vi "一体站流程质控自动启动.vi"(6 "CODMn量程切换":enum32{"H", "L", "AUTO"}(ring)=enum."AUTO", 8 "总磷量程切换":enum32{"H", "L", "AUTO"}(ring)=enum."AUTO", 9 "总氮量程切换":enum32{"H", "L", "AUTO"}(ring)=enum."AUTO", 10 "氨氮量程切换":enum32{"H", "L", "AUTO"}(ring)=enum."AUTO", 11 "参数":T1={"是否启用仪器"=FALSE, "CODMn"={"启动测量模式"={"测量模式"=enum."水样测量"}, "确定按钮"=TRUE}, "启动模块"={"氨氮"=FALSE, "总磷"=FALSE, "总氮"=FALSE, "CODMn"=FALSE, "CODCr"=FALSE}, "常规启动"=FALSE, "直接启动"=FALSE}) -> ()   [LabVIEW 2016, in "质控单元.lvlib"]
panel:
  out "枚举 2":enum16{"初始化", "采配水启动", "等待", "配水", "排水", "结束"}(ring)
  out "枚举":enum16{"初始化", "采配水启动", "等待", "配水", "排水", "结束"}(ring)
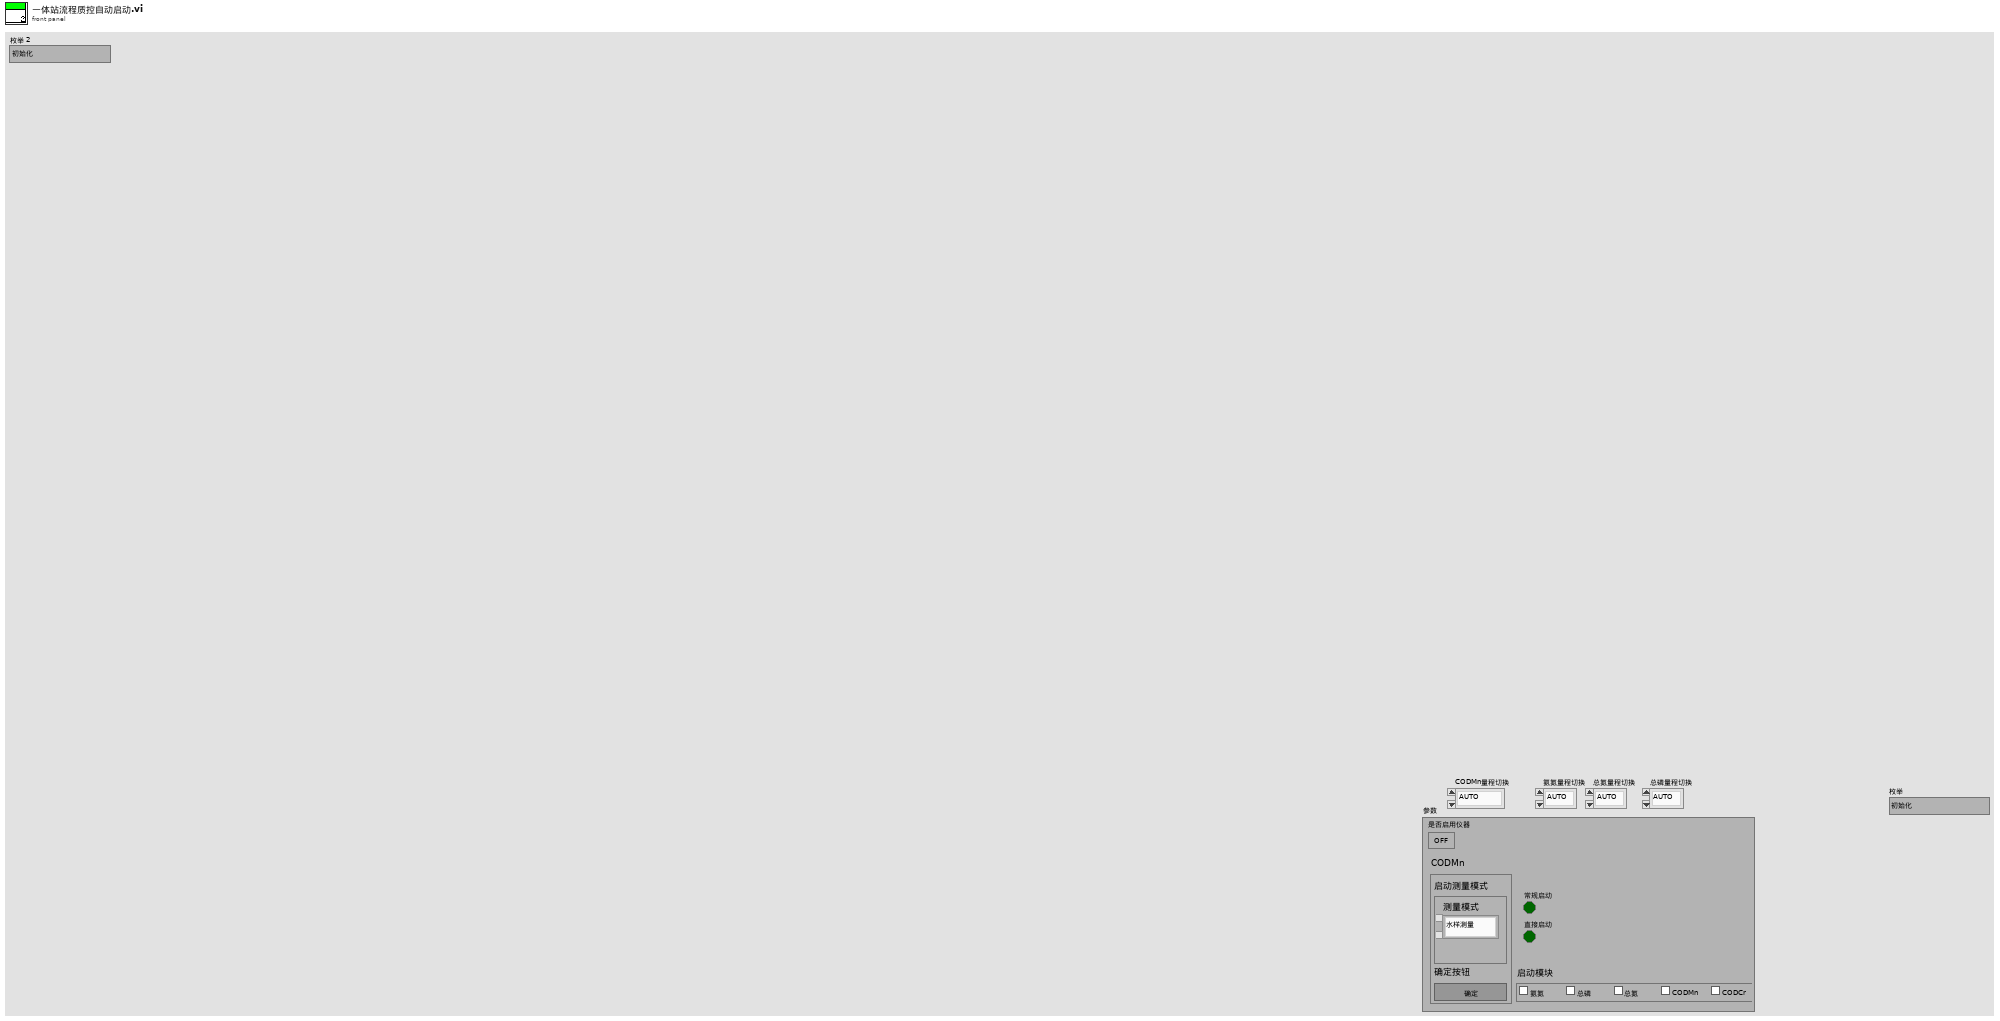
[diagram p1: front panel]
types:
  T1 = cluster{"是否启用仪器":bool, "CODMn":cluster{"启动测量模式":cluster{"测量模式":enum16{"水样测量", "标样核查", "加标回收", "平行样", "校零", "校标"}}, "确定按钮":bool}, "启动模块":cluster{"氨氮":bool, "总磷":bool, "总氮":bool, "CODMn":bool, "CODCr":bool}, "常规启动":bool, "直接启动":bool}
  T2 = cluster{"命令":string, cluster{"starting address":u16, "holding register value":u16}}
  T3 = cluster{"R0":i16, "R1":i16, "R2":i16, "R3":i16, "R4":i16, "R5":i16, "R6":i16, "R7":i16, "R8":i16, "R9":i16, "R10":i16, "R11":i16, "R12":i16, "R13":i16, "R14":i16, "R15":i16, "R16":i16, "R17":i16, "R18":i16, "R19":i16, "R20":i16, "R21":i16, "R22":i16, "R23":i16, "R24":i16, "R25":i16, "R26":i16, "R27":i16, "R28":i16, "R29":i16, "R30":i16, "R31":i16, "R32":i16, "R33":i16, "R34":i16, "R35":i16, "R36":i16, "R37":i16, "R38":i16, "R39":i16, "R40":i16, "R41":i16, "R42":i16, "R43":i16, "R44":i16, "R45":i16, "R46":i16, "R47":i16, "R48":i16, "R49":i16, "R50":i16, "R51":i16, "R52":i16, "R53":i16, "R54":i16, "R55":i16, "R56":i16}
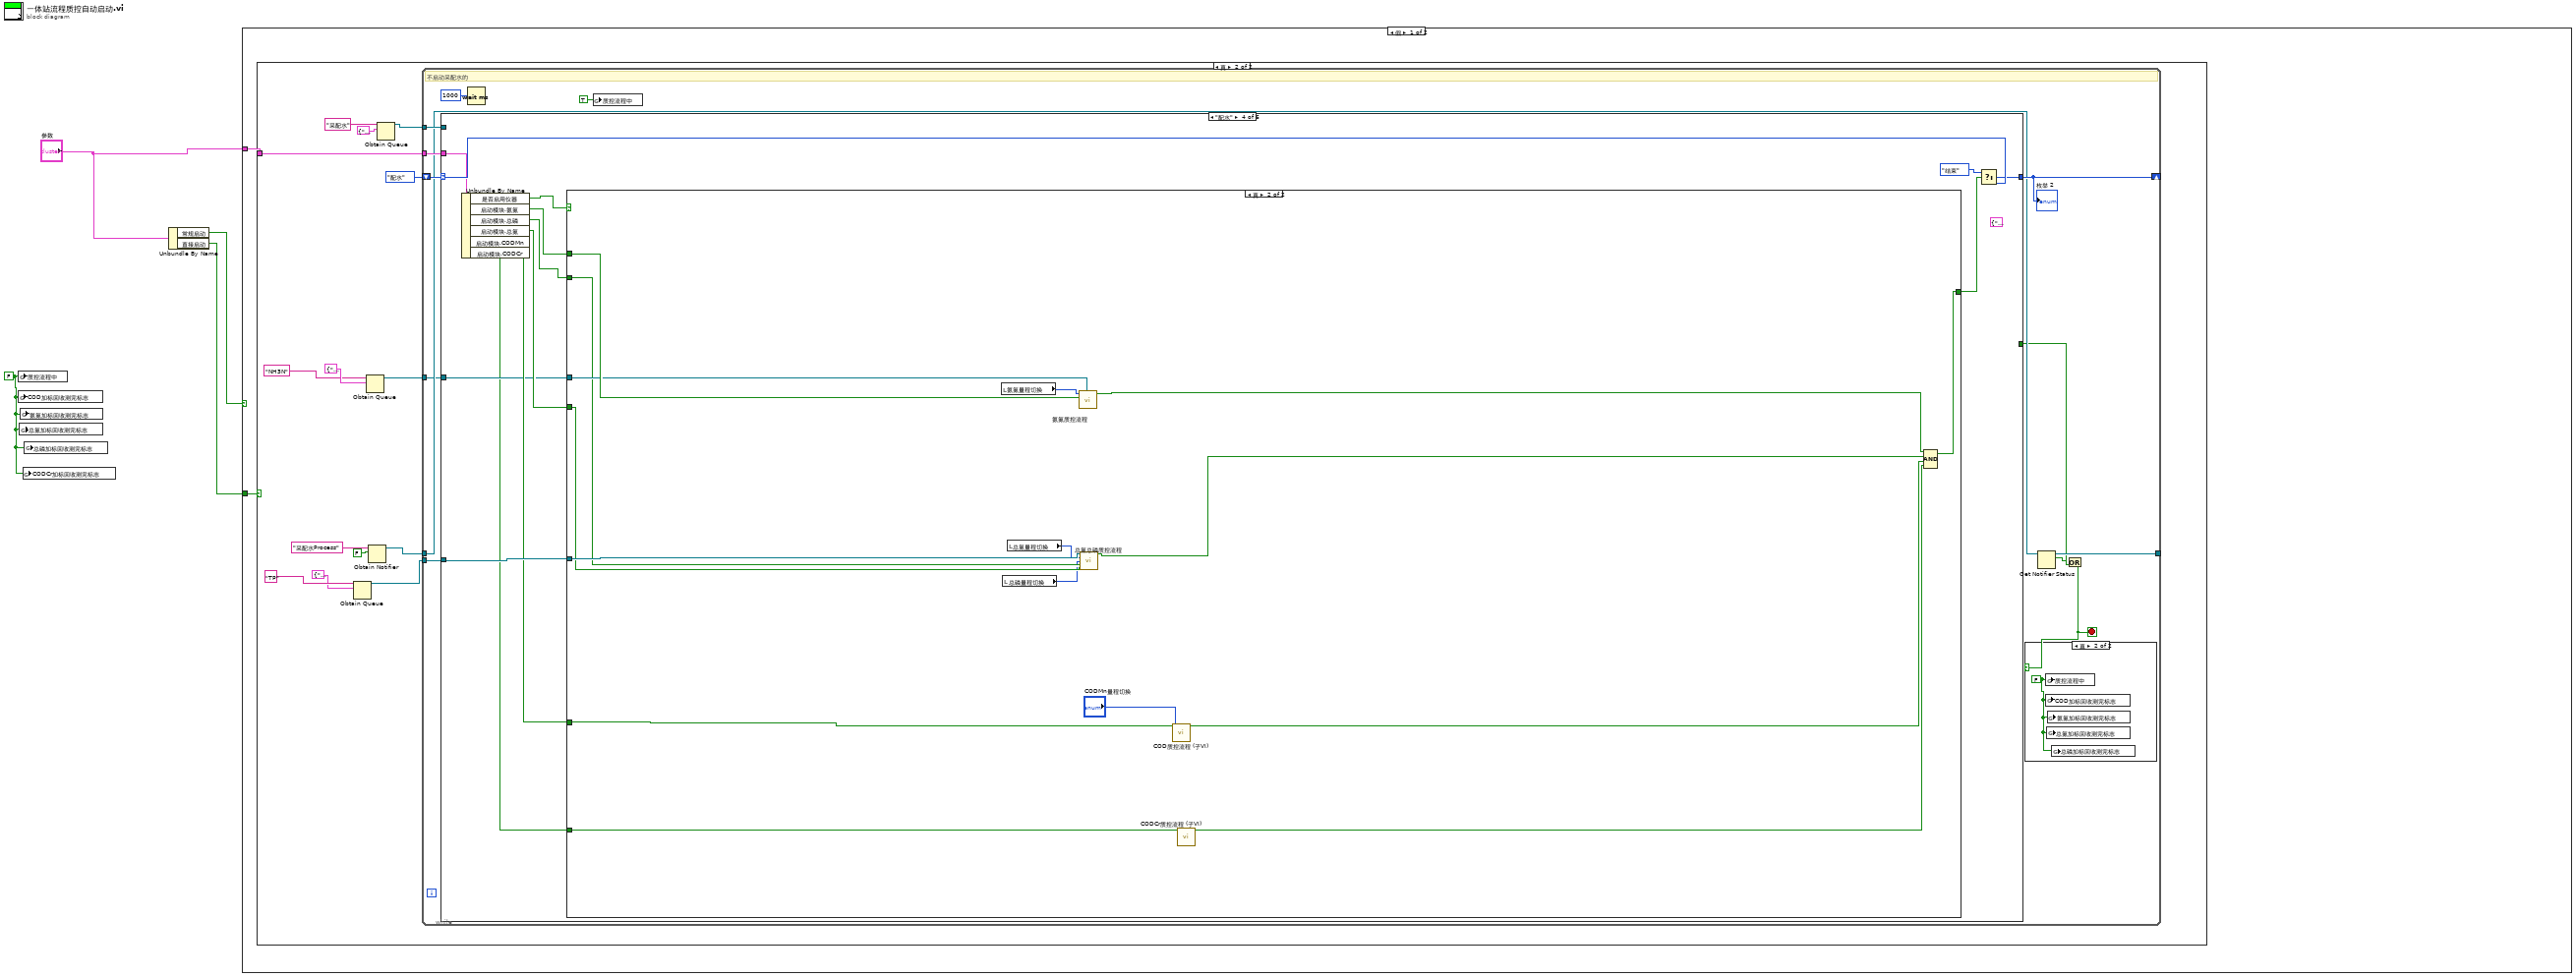
[diagram p0: block diagram]
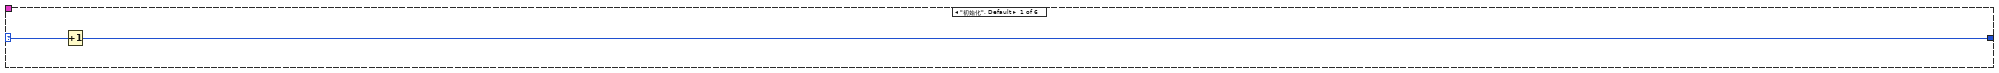
[diagram p4: hidden frame]
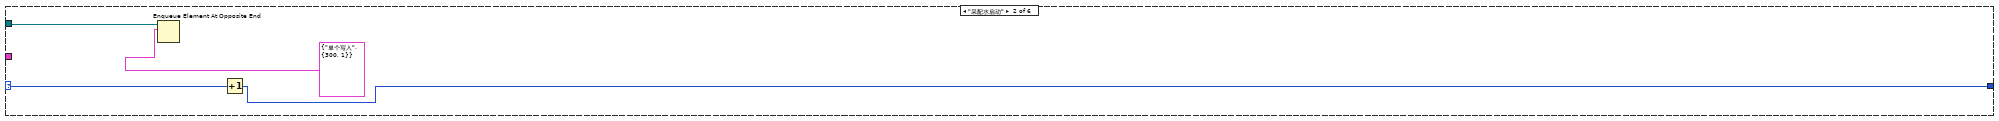
[diagram p5: hidden frame]
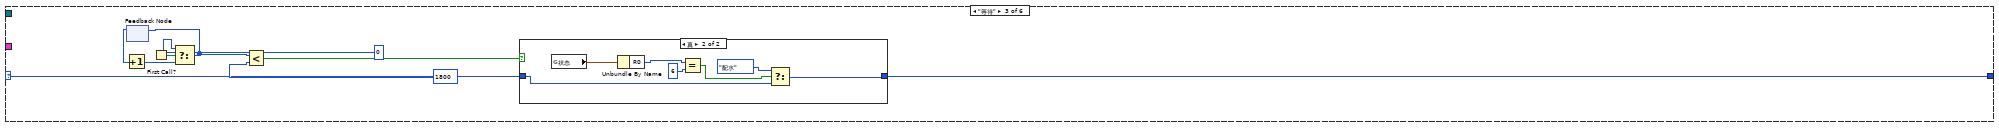
[diagram p6: hidden frame]
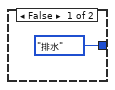
[diagram p7: hidden frame]
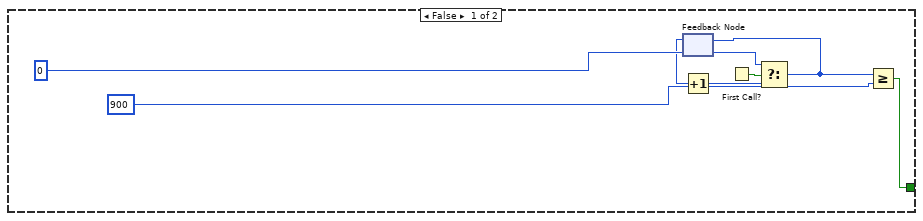
[diagram p8: hidden frame]
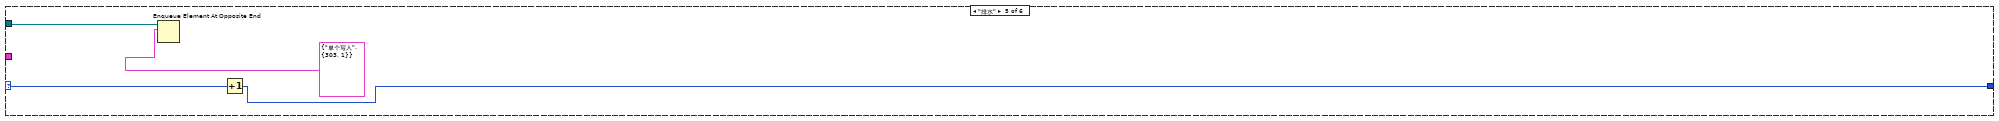
[diagram p9: hidden frame]
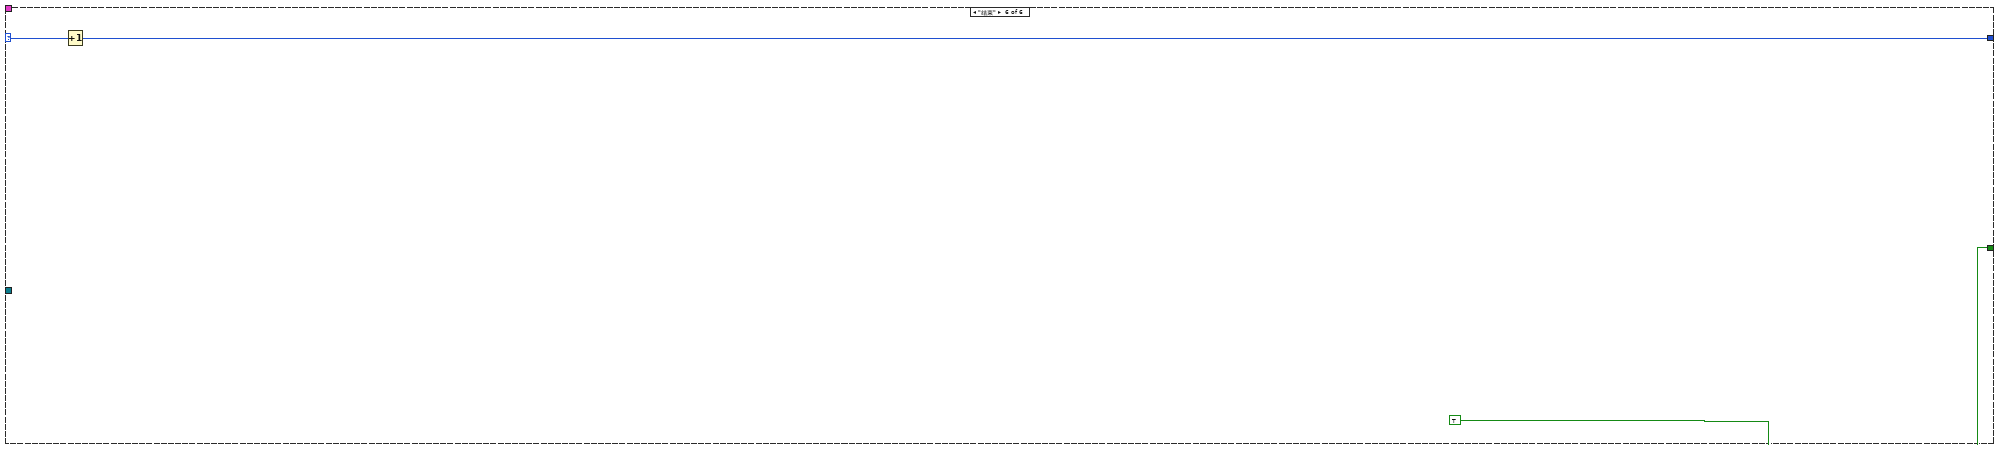
[diagram p10: hidden frame]
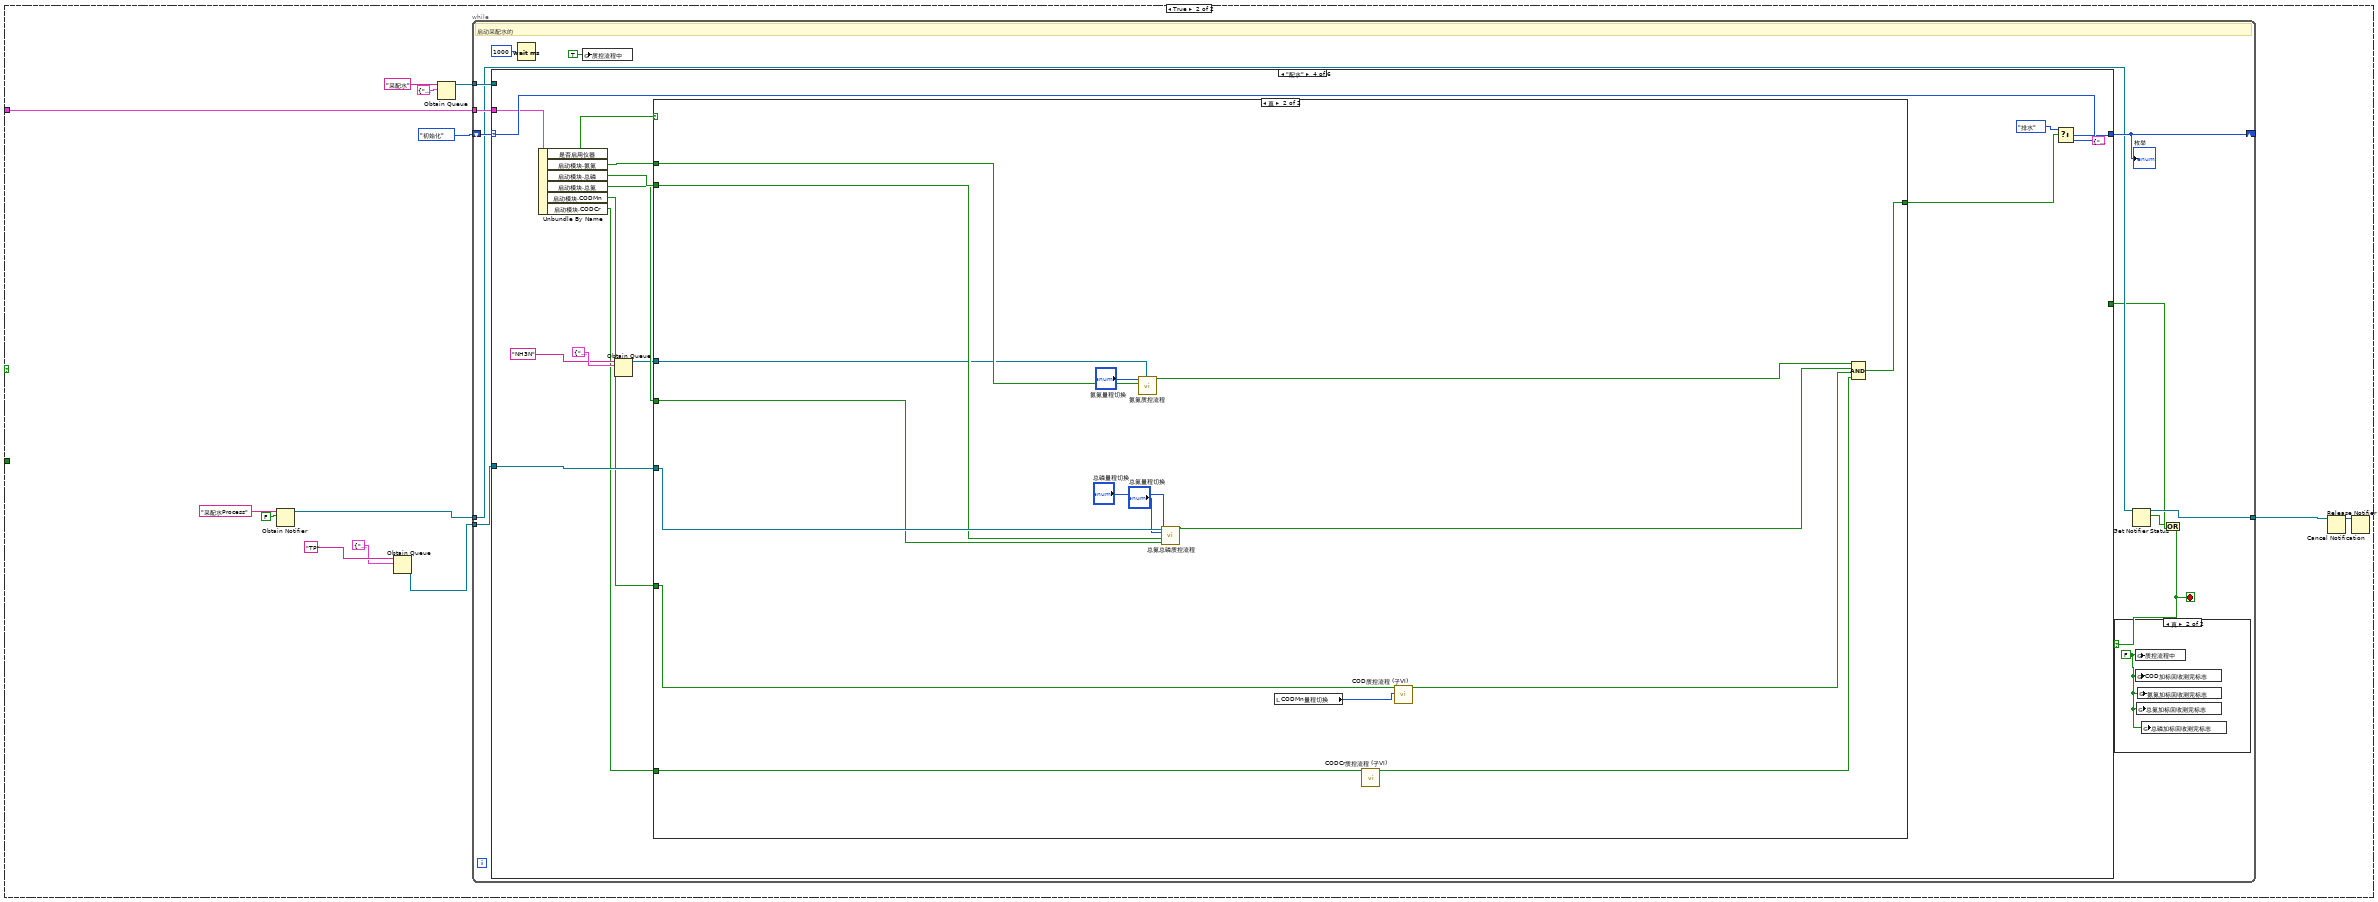
[diagram p11: hidden frame]
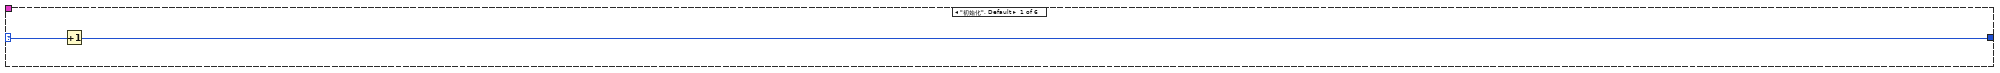
[diagram p13: hidden frame]
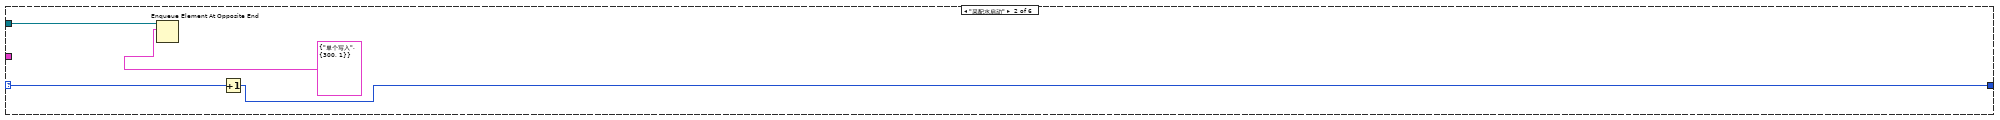
[diagram p14: hidden frame]
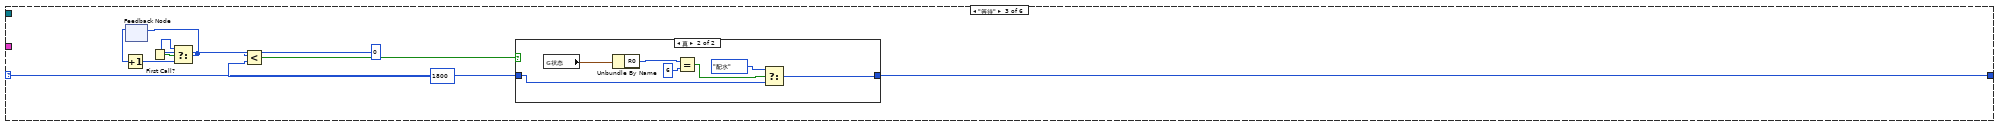
[diagram p15: hidden frame]
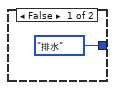
[diagram p16: hidden frame]
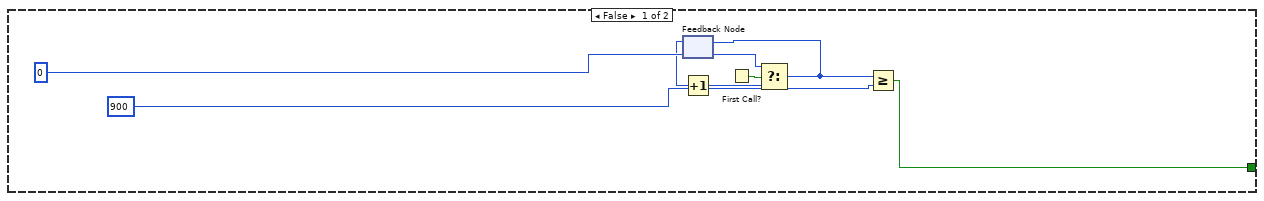
[diagram p17: hidden frame]
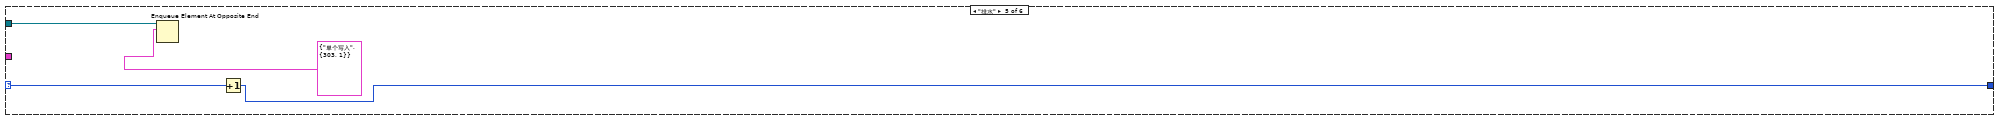
[diagram p18: hidden frame]
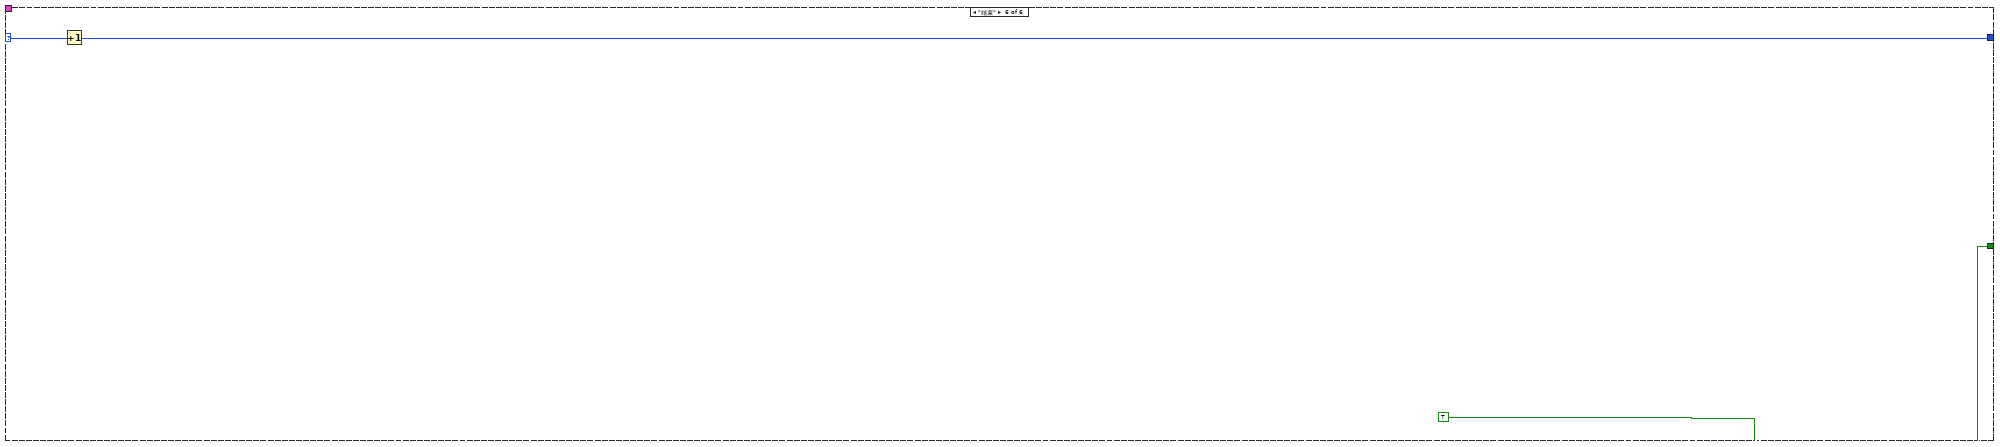
[diagram p19: hidden frame]
diagram:
  w1 = FALSE ("质控流程中")
  n1 = global write "质控测完标志全局 1.vi" "质控流程中"(w1) -> ()
  n2 = global write "质控测完标志全局 1.vi" "COD加标回收测完标志"(w1) -> ()
  n3 = global write "质控测完标志全局 1.vi" "总氮加标回收测完标志"(w1) -> ()
  n4 = global write "质控测完标志全局 1.vi" "氨氮加标回收测完标志"(w1) -> ()
  n5 = global write "质控测完标志全局 1.vi" "CODCr加标回收测完标志"(w1) -> ()
  n6 = global write "质控测完标志全局 1.vi" "总磷加标回收测完标志"(w1) -> ()
  n7 = Unbundle By Name("参数") -> ("常规启动"=w3:bool, "直接启动"=w2:bool)
  n8 = case shown="假" w3 {
    tunnel: "参数" -> [w5 w101]
    tunnel: w2 -> [w6 _]
    frame False {
      n9 = case shown="真" w6 {
        tunnel: w5 -> [_ w19]
        frame False {
        }
        frame True {
          n10 = Obtain Queue(name (unnamed)="TP" ("名称（未命名）"), element data type=cluster{"命令":string, "data":variant} {"命令"="", "data"=variant}) -> (queue out=w10:refnum<queue>)  [unwired: 3 in, 2 out]
          n11 = Obtain Queue(name (unnamed)="NH3N" ("名称（未命名）"), element data type=cluster{"命令":string, "data":variant} {"命令"="", "data"=variant}) -> (queue out=w7:refnum<queue>)  [unwired: 3 in, 2 out]
          n12 = Obtain Notifier(name (unnamed)="采配水Process" ("名称（未命名）"), notification data type=FALSE) -> (notifier out=w13:refnum<notifier>)  [unwired: 2 in, 2 out]
          n13 = Obtain Queue(name (unnamed)="采配水" ("名称（未命名）"), element data type=cluster{"命令":string, "数据":variant} {"命令"="", "数据"=variant}) -> (queue out=w16:refnum<queue>)  [unwired: 3 in, 2 out]
          n14 = while {
            tunnel: w16 -> [w33]
            shift-right: [w31] -> _
            shift-left: enum16{"初始化", "采配水启动", "等待", "配水", "排水", "结束"}."配水" ("枚举") -> [w32]
            tunnel: w10 -> [w29]
            tunnel: w19 -> [w28]
            tunnel: w13 -> [w27]
            tunnel: [w26] -> _
            tunnel: w7 -> [w23]
            stop <- w22 stop-if-true
            # "不启动采配水的"
            n15 = case shown="\"配水\"" w32 {
              selector: w32 -> [w36 w38 w47 w69 w95 w100]
              tunnel: w33 -> [_ w39 _ _ w96 _]
              tunnel: [w35 w37 w46 w68 w94 w99] -> w31
              tunnel: [_ _ _ _ _ TRUE] -> w25
              tunnel: w29 -> [_ _ _ w67 _ _]
              tunnel: w28 -> [_ _ _ w64 _ _]
              tunnel: w23 -> [_ _ _ w59 _ _]
              frame "初始化", Default {
                n16 = Increment(x=w36) -> (x+1=w35:enum16{"初始化", "采配水启动", "等待", "配水", "排水", "结束"})
              }
              frame "采配水启动" {
                n17 = Enqueue Element At Opposite End(queue=w39, element=T2 {"命令"="单个写入", {"starting address"=300, "holding register value"=1}} ("元素")) -> ()  [unwired: 2 in, 3 out]
                n18 = Increment(x=w38) -> (x+1=w37:enum16{"初始化", "采配水启动", "等待", "配水", "排水", "结束"})
              }
              frame "等待" {
                n19 = feedback #1() -> (w43:i32)  [unwired: 1 in]
                n20 = Increment(x=w43) -> (x+1=w42:i32)
                n21 = First Call?() -> (First Call?: T/F=w44:bool)
                n22 = Select(t=0, s=w44, f=w42) -> (s? t:f=w41:i32)
                n23 = feedback-in #1(w41) -> ()
                n24 = Less?(x=w41, y=1800) -> (x < y?=w48:bool)
                n25 = case shown="真" w48 {
                  tunnel: w47 -> [_ w53]
                  tunnel: [enum16{"初始化", "采配水启动", "等待", "配水", "排水", "结束"}."排水" ("枚举") w52] -> w46
                  frame False {
                  }
                  frame True {
                    n26 = global read "与采配水交互全局.vi" "状态"() -> (w51:T3)
                    n27 = Unbundle By Name(w51) -> ("R0"=w57:i16)
                    n28 = Equal?(x=w57, y=i16 6) -> (x = y?=w55:bool)
                    n29 = Select(t=enum16{"初始化", "采配水启动", "等待", "配水", "排水", "结束"}."配水" ("枚举"), s=w55, f=w53) -> (s? t:f=w52:enum16{"初始化", "采配水启动", "等待", "配水", "排水", "结束"})
                  }
                }
              }
              frame "配水" {
                (unwired) cluster{"命令":string, "data":variant} {"命令"="启动", "data"=variant(cluster{"站号":u16, "控制命令输出":u16[]} {"站号"=1, "控制命令输出"=[256, 0]})} ("元素")
                n30 = Unbundle By Name(w64) -> ("是否启用仪器"=w66:bool, "启动模块.氨氮"=w62:bool, "启动模块.总磷"=w63:bool, "启动模块.总氮"=w60:bool, "启动模块.CODMn"=w61:bool, "启动模块.CODCr"=w58:bool)
                n31 = case shown="真" w66 {
                  tunnel: w67 -> [_ w87]
                  tunnel: [w71 w93] -> w65
                  tunnel: w63 -> [_ w86]
                  tunnel: w62 -> [_ w92]
                  tunnel: w61 -> [_ w91]
                  tunnel: w60 -> [_ w85]
                  tunnel: w59 -> [_ w89]
                  tunnel: w58 -> [_ w79]
                  frame False {
                    n32 = feedback #2() -> (w75:i32)  [unwired: 1 in]
                    n33 = Increment(x=w75) -> (x+1=w74:i32)
                    n34 = First Call?() -> (First Call?: T/F=w76:bool)
                    n35 = Select(t=0, s=w76, f=w74) -> (s? t:f=w72:i32)
                    n36 = feedback-in #2(w72) -> ()
                    n37 = Greater Or Equal?(x=w72, y=900) -> (x >= y?=w71:bool)
                  }
                  frame True {
                    n38 = local read "氨氮量程切换"() -> (w80:enum32{"H", "L", "AUTO"})
                    n39 = local read "总磷量程切换"() -> (w82:enum32{"H", "L", "AUTO"})
                    n40 = local read "总氮量程切换"() -> (w81:enum32{"H", "L", "AUTO"})
                    n41 = call "氨氮质控流程.vi"("队列输入NH3"=w89, "氨氮"=w92, "氨氮量程切换"=w80) -> ("布尔"=w90:bool)  [unwired: 7 in, 1 out]
                    n42 = call "总氮总磷质控流程.vi"("队列输入TP"=w87, "总氮量程切换"=w81, "总磷量程切换"=w82, "总磷"=w86, "总氮"=w85) -> ("布尔"=w84:bool)  [unwired: 8 in, 2 out]
                    n43 = call "COD质控流程 (子VI).vi"("CODMn量程切换"="CODMn量程切换", "COD"=w91) -> ("布尔"=w88:bool)  [unwired: 8 in, 1 out]
                    n44 = call "CODCr质控流程 (子VI).vi"("CODCr"=w79) -> ("布尔"=w78:bool)  [unwired: 9 in, 1 out]
                    n45 = Compound Arithmetic op=AND ("复合运算")(w90, w84, w88, w78) -> (w93:bool)
                  }
                }
                n46 = Select(t=enum16{"初始化", "采配水启动", "等待", "配水", "排水", "结束"}."结束" ("枚举"), s=w65, f=w69) -> (s? t:f=w68:enum16{"初始化", "采配水启动", "等待", "配水", "排水", "结束"})
              }
              frame "排水" {
                n47 = Enqueue Element At Opposite End(queue=w96, element=T2 {"命令"="单个写入", {"starting address"=303, "holding register value"=1}} ("元素")) -> ()  [unwired: 2 in, 3 out]
                n48 = Increment(x=w95) -> (x+1=w94:enum16{"初始化", "采配水启动", "等待", "配水", "排水", "结束"})
              }
              frame "结束" {
                n49 = Increment(x=w100) -> (x+1=w99:enum16{"初始化", "采配水启动", "等待", "配水", "排水", "结束"})
              }
            }
            "枚举 2" <- w31
            n50 = Wait (ms)(milliseconds to wait=u32 1000 ("等待时间（毫秒）")) -> ()  [unwired: 1 out]
            n51 = global write "质控测完标志全局 1.vi" "质控流程中"(TRUE ("质控流程中")) -> ()
            n52 = Get Notifier Status(notifier=w27) -> (notifier out=w26:refnum<notifier>, current notification=w24:bool)  [unwired: 1 in, 3 out]
            n53 = Or(x=w24, y=w25) -> (x .or. y?=w22:bool)
            n54 = case shown="真" w22 {
              frame False {
              }
              frame True {
                w34 = FALSE ("质控流程中")
                n55 = global write "质控测完标志全局 1.vi" "质控流程中"(w34) -> ()
                n56 = global write "质控测完标志全局 1.vi" "COD加标回收测完标志"(w34) -> ()
                n57 = global write "质控测完标志全局 1.vi" "总氮加标回收测完标志"(w34) -> ()
                n58 = global write "质控测完标志全局 1.vi" "氨氮加标回收测完标志"(w34) -> ()
                n59 = global write "质控测完标志全局 1.vi" "总磷加标回收测完标志"(w34) -> ()
              }
            }
          }
        }
      }
    }
    frame True {
      n60 = Obtain Notifier(name (unnamed)="采配水Process" ("名称（未命名）"), notification data type=FALSE) -> (notifier out=w104:refnum<notifier>)  [unwired: 2 in, 2 out]
      n61 = Obtain Queue(name (unnamed)="TP" ("名称（未命名）"), element data type=cluster{"命令":string, "data":variant} {"命令"="", "data"=variant}) -> (queue out=w107:refnum<queue>)  [unwired: 3 in, 2 out]
      n62 = Obtain Queue(name (unnamed)="采配水" ("名称（未命名）"), element data type=cluster{"命令":string, "数据":variant} {"命令"="", "数据"=variant}) -> (queue out=w111:refnum<queue>)  [unwired: 3 in, 2 out]
      n63 = while {
        tunnel: w111 -> [w125]
        shift-right: [w123] -> _
        shift-left: enum16{"初始化", "采配水启动", "等待", "配水", "排水", "结束"}."初始化" ("枚举") -> [w124]
        tunnel: w107 -> [w121]
        tunnel: w101 -> [w120]
        tunnel: w104 -> [w119]
        tunnel: [w118] -> w103
        stop <- w115 stop-if-true
        # "启动采配水的"
        n64 = case shown="\"配水\"" w124 {
          selector: w124 -> [w128 w130 w139 w163 w189 w194]
          tunnel: w125 -> [_ w131 _ _ w190 _]
          tunnel: [w127 w129 w138 w162 w188 w193] -> w123
          tunnel: [_ _ _ _ _ TRUE] -> w117
          tunnel: w121 -> [_ _ _ w161 _ _]
          tunnel: w120 -> [_ _ _ w158 _ _]
          frame "初始化", Default {
            n65 = Increment(x=w128) -> (x+1=w127:enum16{"初始化", "采配水启动", "等待", "配水", "排水", "结束"})
          }
          frame "采配水启动" {
            n66 = Enqueue Element At Opposite End(queue=w131, element=T2 {"命令"="单个写入", {"starting address"=300, "holding register value"=1}} ("元素")) -> ()  [unwired: 2 in, 3 out]
            n67 = Increment(x=w130) -> (x+1=w129:enum16{"初始化", "采配水启动", "等待", "配水", "排水", "结束"})
          }
          frame "等待" {
            n68 = feedback #3() -> (w135:i32)  [unwired: 1 in]
            n69 = Increment(x=w135) -> (x+1=w134:i32)
            n70 = First Call?() -> (First Call?: T/F=w136:bool)
            n71 = Select(t=0, s=w136, f=w134) -> (s? t:f=w133:i32)
            n72 = feedback-in #3(w133) -> ()
            n73 = Less?(x=w133, y=1800) -> (x < y?=w140:bool)
            n74 = case shown="真" w140 {
              tunnel: w139 -> [_ w145]
              tunnel: [enum16{"初始化", "采配水启动", "等待", "配水", "排水", "结束"}."排水" ("枚举") w144] -> w138
              frame False {
              }
              frame True {
                n75 = global read "与采配水交互全局.vi" "状态"() -> (w143:T3)
                n76 = Unbundle By Name(w143) -> ("R0"=w149:i16)
                n77 = Equal?(x=w149, y=i16 6) -> (x = y?=w147:bool)
                n78 = Select(t=enum16{"初始化", "采配水启动", "等待", "配水", "排水", "结束"}."配水" ("枚举"), s=w147, f=w145) -> (s? t:f=w144:enum16{"初始化", "采配水启动", "等待", "配水", "排水", "结束"})
              }
            }
          }
          frame "配水" {
            (unwired) cluster{"命令":string, "data":variant} {"命令"="启动", "data"=variant(cluster{"站号":u16, "控制命令输出":u16[]} {"站号"=1, "控制命令输出"=[256, 0]})} ("元素")
            n79 = Unbundle By Name(w158) -> ("是否启用仪器"=w160:bool, "启动模块.氨氮"=w156:bool, "启动模块.总磷"=w157:bool, "启动模块.总氮"=w154:bool, "启动模块.CODMn"=w155:bool, "启动模块.CODCr"=w150:bool)
            n80 = Obtain Queue(name (unnamed)="NH3N" ("名称（未命名）"), element data type=cluster{"命令":string, "data":variant} {"命令"="", "data"=variant}) -> (queue out=w151:refnum<queue>)  [unwired: 3 in, 2 out]
            n81 = case shown="真" w160 {
              tunnel: w161 -> [_ w182]
              tunnel: [w165 w186] -> w159
              tunnel: w157 -> [_ w181]
              tunnel: w156 -> [_ w185]
              tunnel: w155 -> [_ w184]
              tunnel: w154 -> [_ w180]
              tunnel: w151 -> [_ w178]
              tunnel: w150 -> [_ w173]
              frame False {
                n82 = feedback #4() -> (w169:i32)  [unwired: 1 in]
                n83 = Increment(x=w169) -> (x+1=w168:i32)
                n84 = First Call?() -> (First Call?: T/F=w170:bool)
                n85 = Select(t=0, s=w170, f=w168) -> (s? t:f=w166:i32)
                n86 = feedback-in #4(w166) -> ()
                n87 = Greater Or Equal?(x=w166, y=900) -> (x >= y?=w165:bool)
              }
              frame True {
                n88 = call "氨氮质控流程.vi"("队列输入NH3"=w178, "氨氮"=w185, "氨氮量程切换"="氨氮量程切换") -> ("布尔"=w187:bool)  [unwired: 7 in, 1 out]
                n89 = call "总氮总磷质控流程.vi"("队列输入TP"=w182, "总氮量程切换"="总氮量程切换", "总磷量程切换"="总磷量程切换", "总磷"=w181, "总氮"=w180) -> ("布尔"=w179:bool)  [unwired: 8 in, 2 out]
                n90 = local read "CODMn量程切换"() -> (w177:enum32{"H", "L", "AUTO"})
                n91 = call "CODCr质控流程 (子VI).vi"("CODCr"=w173) -> ("布尔"=w172:bool)  [unwired: 9 in, 1 out]
                n92 = call "COD质控流程 (子VI).vi"("CODMn量程切换"=w177, "COD"=w184) -> ("布尔"=w183:bool)  [unwired: 8 in, 1 out]
                n93 = Compound Arithmetic op=AND ("复合运算")(w187, w179, w183, w172) -> (w186:bool)
              }
            }
            n94 = Select(t=enum16{"初始化", "采配水启动", "等待", "配水", "排水", "结束"}."排水" ("枚举"), s=w159, f=w163) -> (s? t:f=w162:enum16{"初始化", "采配水启动", "等待", "配水", "排水", "结束"})
          }
          frame "排水" {
            n95 = Enqueue Element At Opposite End(queue=w190, element=T2 {"命令"="单个写入", {"starting address"=303, "holding register value"=1}} ("元素")) -> ()  [unwired: 2 in, 3 out]
            n96 = Increment(x=w189) -> (x+1=w188:enum16{"初始化", "采配水启动", "等待", "配水", "排水", "结束"})
          }
          frame "结束" {
            n97 = Increment(x=w194) -> (x+1=w193:enum16{"初始化", "采配水启动", "等待", "配水", "排水", "结束"})
          }
        }
        "枚举" <- w123
        n98 = Wait (ms)(milliseconds to wait=u32 1000 ("等待时间（毫秒）")) -> ()  [unwired: 1 out]
        n99 = global write "质控测完标志全局 1.vi" "质控流程中"(TRUE ("质控流程中")) -> ()
        n100 = Get Notifier Status(notifier=w119) -> (notifier out=w118:refnum<notifier>, current notification=w116:bool)  [unwired: 1 in, 3 out]
        n101 = Or(x=w116, y=w117) -> (x .or. y?=w115:bool)
        n102 = case shown="真" w115 {
          frame False {
          }
          frame True {
            w126 = FALSE ("质控流程中")
            n103 = global write "质控测完标志全局 1.vi" "质控流程中"(w126) -> ()
            n104 = global write "质控测完标志全局 1.vi" "COD加标回收测完标志"(w126) -> ()
            n105 = global write "质控测完标志全局 1.vi" "总氮加标回收测完标志"(w126) -> ()
            n106 = global write "质控测完标志全局 1.vi" "氨氮加标回收测完标志"(w126) -> ()
            n107 = global write "质控测完标志全局 1.vi" "总磷加标回收测完标志"(w126) -> ()
          }
        }
      }
      n108 = Cancel Notification(0:w103) -> (8:w102:refnum<notifier>)  [unwired: 1 in, 2 out]
      n109 = Release Notifier(notifier=w102) -> ()  [unwired: 2 in, 3 out]
    }
  }
